vi "Real time monitoring.vi"() -> ()   [LabVIEW 2013]
uses:
  <vilib>/Instr/_visa.llb/VISA Configure Serial Port (Instr).vi
panel:
  in  "Stop":bool
  in  "Enter Interval Time":dbl
  in  "Enum":T1(ring)
  out "error out 7":errorcluster
  out "return code":i32
  out "standard error":string
  out "standard output":string
  out "Plot":T2(graph)
  out "error out 6":errorcluster
  in  "File Directory":path
  in  "Baud Rate":u32=9600
  in  "VISA resource name":refnum<visa-resource-name>
  in  "Start":bool
  out "error out 5":errorcluster
  out "read buffer":string
  out "error out 3":errorcluster
  out "error out 2":errorcluster
  in  "Staring Frequency":string
  out "error out":errorcluster
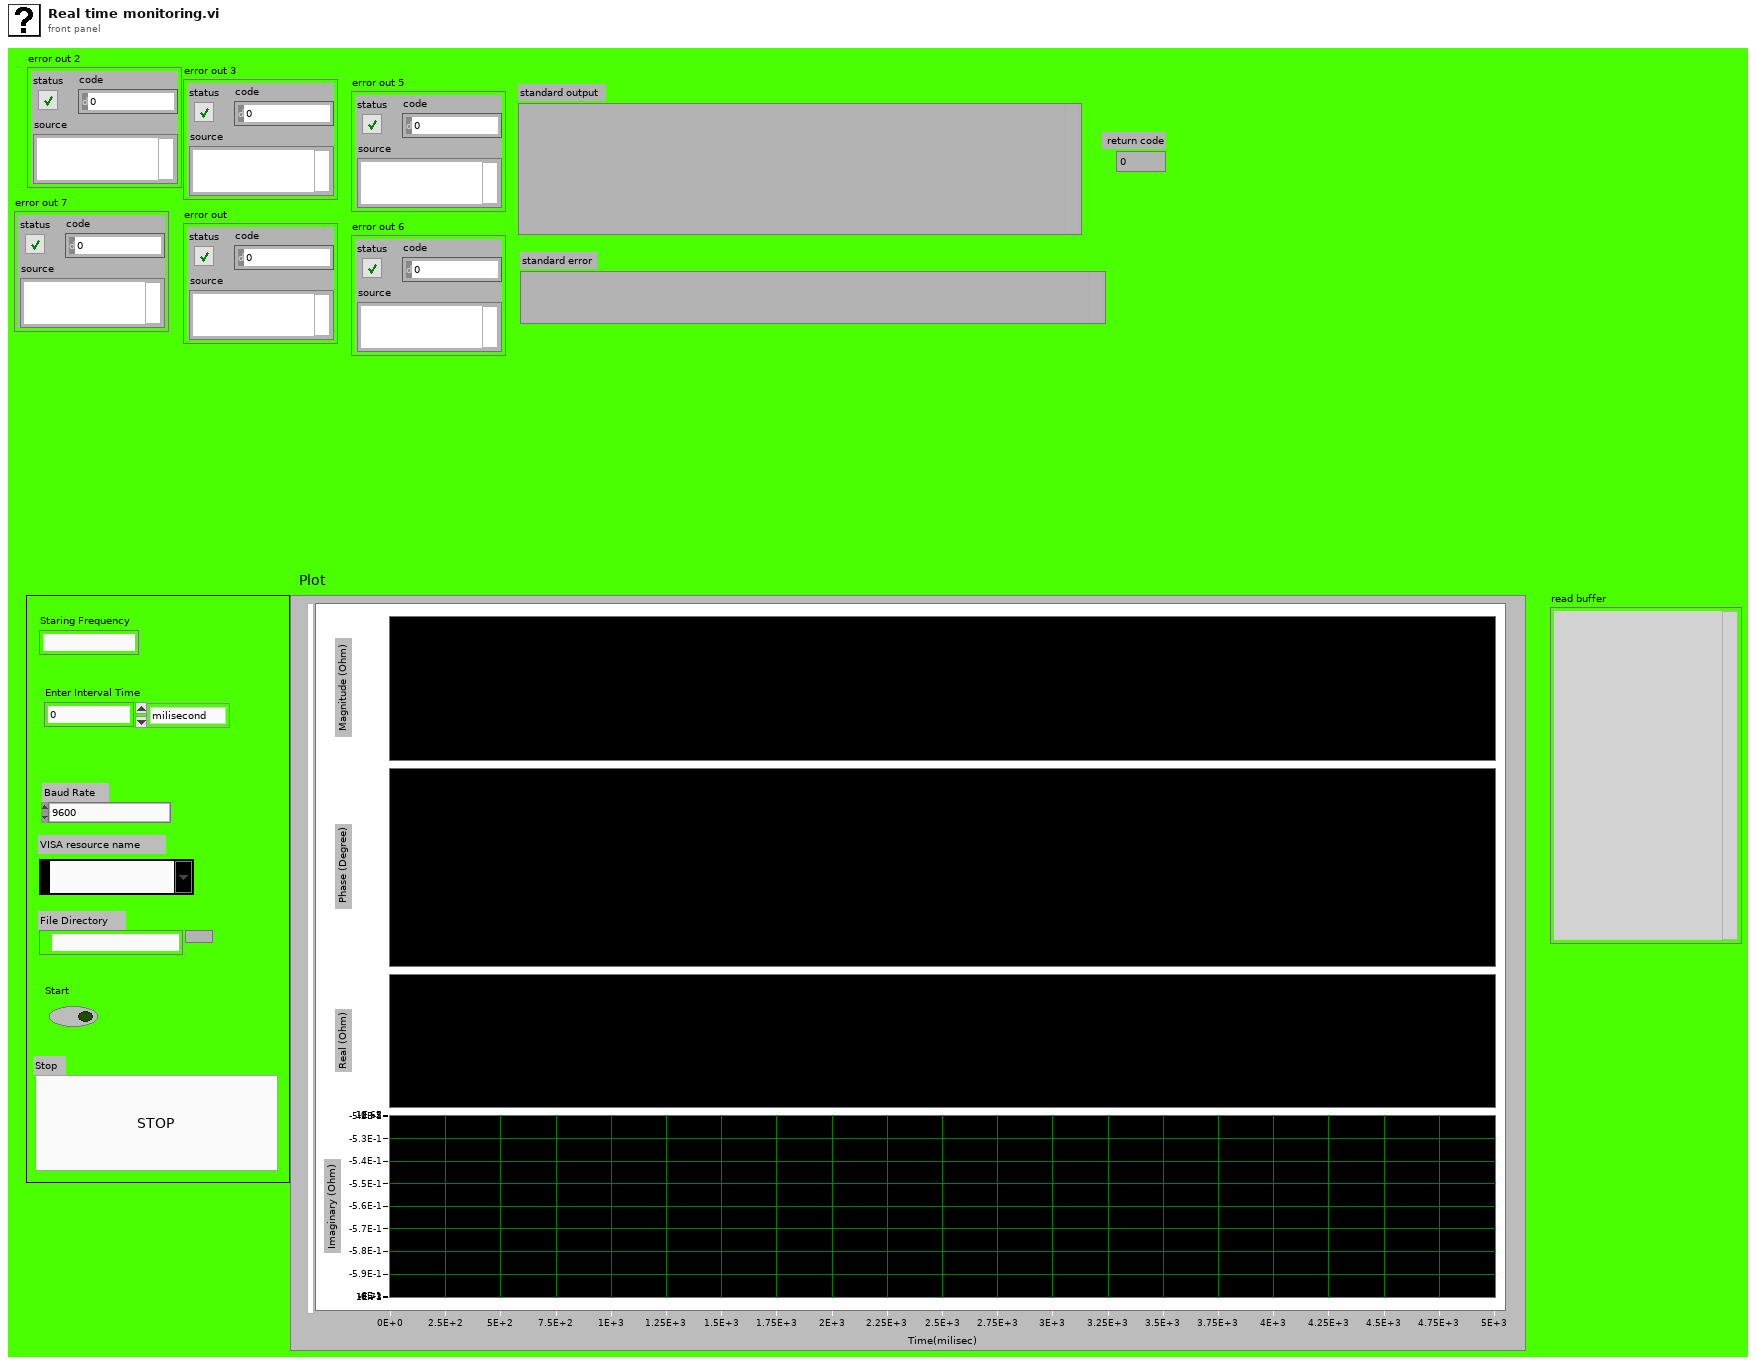
[diagram p1: front panel]
types:
  T1 = enum16{"milisecond", "sec.", "Min.", "Hr.", "Day"}
  T2 = cluster{"array type (2D Dbl)":dbl[], "array type (2D Dbl)":dbl[]}[]
  T3 = cluster{"array type (2D Dbl)":dbl[], "array type (2D Dbl)":dbl[]}
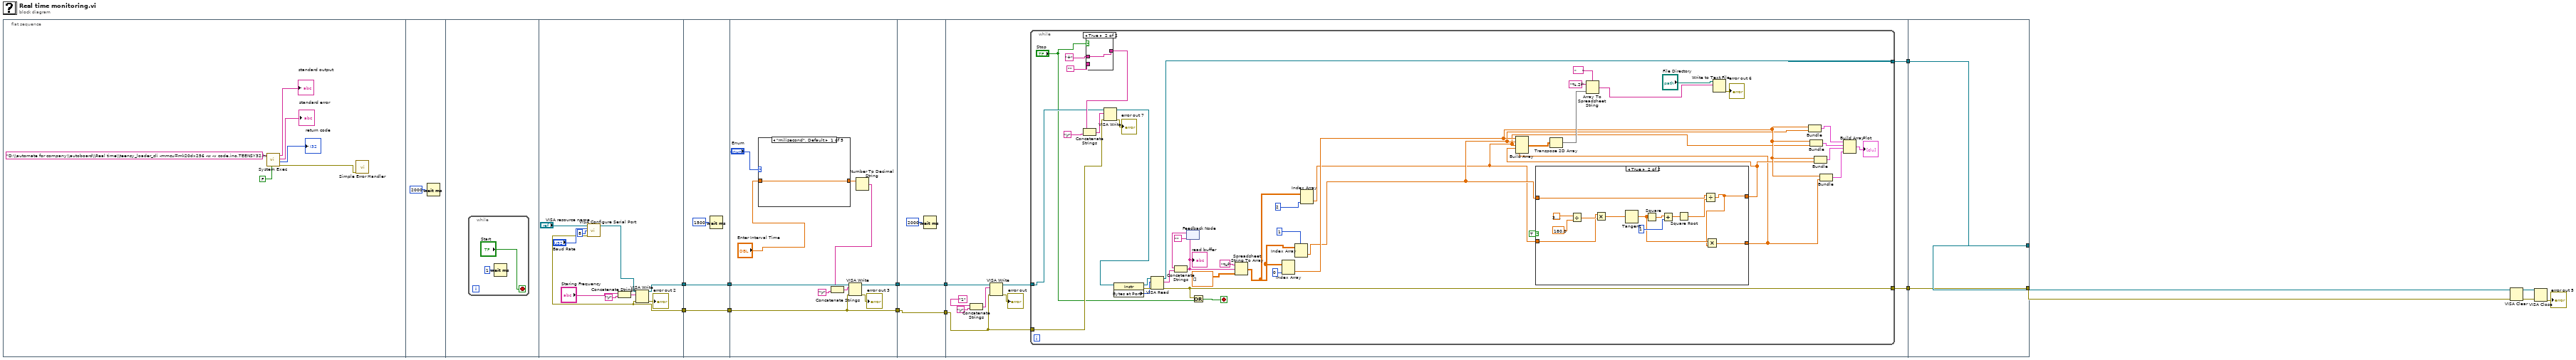
[diagram p0: block diagram]
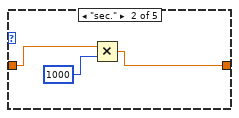
[diagram p2: hidden frame]
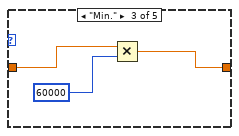
[diagram p3: hidden frame]
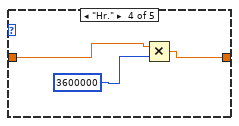
[diagram p4: hidden frame]
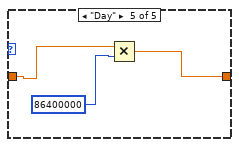
[diagram p5: hidden frame]
diagram:
  n1 = flat-sequence {
    tunnel: [w33] -> w13
    tunnel: [w25] -> w11
    tunnel: w13 -> [w37]
    tunnel: [w37] -> w12
    tunnel: w11 -> [w36]
    tunnel: [w36] -> w10
    tunnel: w12 -> [w44]
    tunnel: [w46] -> w9
    tunnel: w10 -> [w45]
    tunnel: [w45] -> w8
    tunnel: w9 -> [w61]
    tunnel: w8 -> [w62]
    tunnel: [w62] -> w2
    tunnel: [w61] -> w1
    tunnel: [w72] -> w15
    tunnel: [w71] -> w14
    tunnel: w2 -> [w64]
    tunnel: w1 -> [w65]
    tunnel: [w134] -> w7
    tunnel: [w135] -> w6
    tunnel: w15 -> [w135]
    tunnel: w14 -> [w134]
    frame #0 {
      n2 = call <vilib>:"System Exec.vi"("run minimized? (F)"=FALSE, "command line"="D:\\automate for company\\autoboard\\Real time\\teensy_loader_cli -mmcu=mk20dx256 -w -v code.ino.TEENSY32.hex") -> ("error out"=w17:errorcluster, "return code"=→"return code":i32, "standard error"=→"standard error":string, "standard output"=→"standard output":string)  [unwired: 6 in]
      n3 = call <vilib>:"Simple Error Handler.vi"("error in (no error)"=w17) -> ()  [unwired: 1 in, 8 out]
    }
    frame #1 {
      n4 = Wait (ms)(milliseconds to wait=u32 2000) -> ()  [unwired: 1 out]
    }
    frame #2 {
      n5 = while {
        stop <- "Start" stop-if-true
        n6 = Wait (ms)(milliseconds to wait=u32 1 ("대기 시간(ms)")) -> ()  [unwired: 1 out]
      }
    }
    frame #3 {
      n7 = call-poly "VISA Configure Serial Port"("VISA resource name"="VISA resource name", "baud rate (9600)"="Baud Rate", "data bits (8)"=u16 8) -> ("VISA resource name out"=w26:refnum<visa-resource-name>, "error out"=w25:errorcluster)  [unwired: 11 in]
      n8 = Concatenate Strings("Staring Frequency", "\r") -> (w31:string)
      n9 = VISA Write(VISA resource name=w26, write buffer=w31, error in (no error)=w25) -> (VISA resource name out=w33:refnum<visa-resource-name>, error out=→"error out 2":errorcluster)  [unwired: 1 out]
    }
    frame #4 {
      n10 = Wait (ms)(milliseconds to wait=u32 1500) -> ()  [unwired: 1 out]
    }
    frame #5 {
      n11 = case shown="\"milisecond\", Default" "Enum" {
        tunnel: "Enter Interval Time" -> [w48 w50 w54 w55 w60]
        tunnel: [w48 w51 w52 w57 w59] -> w40
        frame "milisecond", Default {
        }
        frame "sec." {
          n12 = Multiply(x=w50, y=1000) -> (x*y=w51:dbl)
        }
        frame "Min." {
          n13 = Multiply(x=w54, y=60000) -> (x*y=w52:dbl)
        }
        frame "Hr." {
          n14 = Multiply(x=w55, y=3600000) -> (x*y=w57:dbl)
        }
        frame "Day" {
          n15 = Multiply(x=w60, y=86400000) -> (x*y=w59:dbl)
        }
      }
      n16 = Number To Decimal String(number=w40) -> (decimal integer string=w38:string)  [unwired: 1 in]
      n17 = Concatenate Strings(w38, "\r") -> (w42:string)
      n18 = VISA Write(VISA resource name=w44, write buffer=w42, error in (no error)=w45) -> (VISA resource name out=w46:refnum<visa-resource-name>, error out=→"error out 3":errorcluster)  [unwired: 1 out]
    }
    frame #6 {
      n19 = Wait (ms)(milliseconds to wait=u32 2000) -> ()  [unwired: 1 out]
    }
    frame #7 {
      n20 = Concatenate Strings("1" ("string"), "\r") -> (w67:string)
      n21 = VISA Write(VISA resource name=w65, write buffer=w67, error in (no error)=w64) -> (VISA resource name out=w69:refnum<visa-resource-name>, error out=→"error out":errorcluster)  [unwired: 1 out]
      n22 = while {
        tunnel: [w113] -> w72
        tunnel: [w111] -> w71
        tunnel: w69 -> [w76]
        tunnel: w64 -> [w75]
        stop <- w112 stop-if-true
        n23 = case shown="True" "Stop" {
          tunnel: "+" -> [_ w118]
          tunnel: "" -> [w117 _]
          tunnel: [w117 w118] -> w78
          frame False {
          }
          frame True {
          }
        }
        n24 = Concatenate Strings(w78, "\r") -> (w81:string)
        n25 = VISA Write(VISA resource name=w76, write buffer=w81, error in (no error)=w75) -> (VISA resource name out=w77:refnum<visa-resource-name>, error out=→"error out 7":errorcluster)  [unwired: 1 out]
        n26 = property on="Property Node" class="Instr"(reference=w77) -> (reference out=w115:refnum<visa-resource-name>, error out=w116:errorcluster, "Bytes at Port"=w114:u32)  [unwired: 1 in]
        n27 = VISA Read(VISA resource name=w115, byte count=w114, error in (no error)=w116) -> (VISA resource name out=w113:refnum<visa-resource-name>, read buffer=w108:string, error out=w111:errorcluster)  [unwired: 1 out]
        n28 = feedback #1("") -> (w109:string)
        n29 = Concatenate Strings(w109, w108) -> (w105:string)
        "read buffer" <- w105
        n30 = feedback-in #1(w105) -> ()
        n31 = Or(x=w111, y="Stop") -> (x .or. y?=w112:bool)
        n32 = Spreadsheet String To Array(format string="%f", spreadsheet string=w105, array type (2D Dbl)=dbl[][] []) -> (array=w101:dbl[][])  [unwired: 1 in]
        n33 = Index Array(array=w101, index (col)=0 ("disabled index (col)")) -> (element=w88:dbl[])  [unwired: 1 in]
        n34 = Index Array(array=w101, index (col)=1 ("disabled index (col)")) -> (element=w85:dbl[])  [unwired: 1 in]
        n35 = Index Array(array=w101, index (col)=2 ("disabled index (col)")) -> (element=w84:dbl[])  [unwired: 1 in]
        n36 = case shown="True" TRUE {
          tunnel: w85 -> [w120 w124]
          tunnel: w84 -> [w119 w123]
          tunnel: [w119 w122] -> w86
          tunnel: [w120 w121] -> w87
          frame False {
          }
          frame True {
            n37 = Divide(x=3.141592653589793, y=180.0) -> (x/y=w131:dbl)
            n38 = Multiply(x=w131, y=w123) -> (x*y=w130:dbl[])
            n39 = Tangent(1:w130) -> (0:w125:dbl[])
            n40 = Square(x=w125) -> (x^2=w129:dbl[])
            n41 = Add(x=w129, y=1) -> (x+y=w127:dbl[])
            n42 = Square Root(x=w127) -> (sqrt(x)=w126:dbl[])
            n43 = Divide(x=w124, y=w126) -> (x/y=w121:dbl[])
            n44 = Multiply(x=w125, y=w121) -> (x*y=w122:dbl[])
          }
        }
        n45 = Build Array(w88, w85, w84, w87, w86) -> (w99:dbl[][])
        n46 = Transpose 2D Array(2D array=w99) -> (transposed array=w98:dbl[][])
        n47 = Array To Spreadsheet String(delimiter (Tab)="    ", array=w98, 3:"%.2f" ("format string")) -> (spreadsheet string=w94:string)
        n48 = Write to Text File(file (use dialog)="File Directory", text=w94) -> (error out=→"error out 6":errorcluster)  [unwired: 2 in, 2 out]
        n49 = Bundle("array type (2D Dbl)"=w88, "array type (2D Dbl)"=w85) -> (w92:T3)  [unwired: 1 in]
        n50 = Bundle("array type (2D Dbl)"=w88, "array type (2D Dbl)"=w84) -> (w91:T3)  [unwired: 1 in]
        n51 = Bundle("array type (2D Dbl)"=w88, "array type (2D Dbl)"=w87) -> (w90:T3)  [unwired: 1 in]
        n52 = Bundle("array type (2D Dbl)"=w88, "array type (2D Dbl)"=w86) -> (w89:T3)  [unwired: 1 in]
        n53 = Build Array(w92, w91, w90, w89) -> (→"Plot":T2)
      }
    }
    frame #8 {
    }
  }
  n54 = VISA Clear(VISA resource name=w6, error in (no error)=w7) -> (VISA resource name out=w4:refnum<visa-resource-name>, error out=w5:errorcluster)
  n55 = VISA Close(VISA resource name=w4, error in (no error)=w5) -> (error out=→"error out 5":errorcluster)
